vi "dfd_Calculate Stopband and Passband from Roll-off.vi"(7 "#channel":i32=4, 11 "roll off":dbl format="%.2f") -> (2 "fstop":dbl, 3 "fpass":dbl)   [LabVIEW 2017, in "NI_DigFilter_FilterBank.lvlib"]
uses:
  <vilib>/addons/Digital Filter Design/NI_DigFilter_FilterBank.lvlib
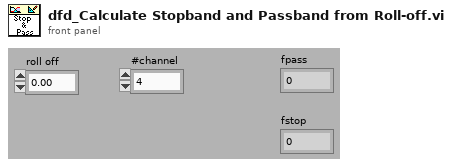
[diagram p1: front panel]
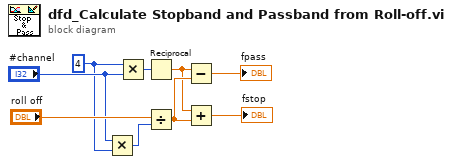
[diagram p0: block diagram]
diagram:
  w4 = 4
  n1 = Multiply(x="#channel", y=w4) -> (x*y=w7:i32)
  n2 = Multiply(x=w4, y="#channel") -> (x*y=w9:i32)
  n3 = Reciprocal(x=w9) -> (1/x=w1:dbl)
  n4 = Divide(x="roll off", y=w7) -> (x/y=w8:dbl)
  n5 = Subtract(x=w1, y=w8) -> (x-y=→"fpass":dbl)
  n6 = Add(x=w1, y=w8) -> (x+y=→"fstop":dbl)
